vi "AIsFIFO.vi"   [LabVIEW 2017]
uses:
  <vilib>/eio/EIONode/EIONode.xnode
  <vilib>/rvi/DataTransferAndStorage/Container/XNode/niFpgaContainer.xnode
  <vilib>/rvi/eio/common/nirviEmuTemplateMethod_errors.vi
  <vilib>/rvi/FIFO/Fifo_Resource/niFpgaFifoEmulationRefIn.vi
diagram:
  n1 = xnode "FPGA I/O Node"() -> ("Mod1/AI0"=w287, "Mod1/AI1"=w284, "Mod1/AI2"=w281, "Mod1/AI3"=w279, "Mod1/AI4"=w275, "Mod1/AI5"=w272, "Mod1/AI6"=w269, "Mod1/AI7"=w266, "Mod1/AI8"=w263, "Mod1/AI9"=w260, "Mod1/AI10"=w257, "Mod1/AI11"=w254, "Mod1/AI12"=w251, "Mod1/AI13"=w248, "Mod1/AI14"=w245, "Mod1/AI15"=w242, "Mod1/AI16"=w239, "Mod1/AI17"=w236, "Mod1/AI18"=w233, "Mod1/AI19"=w230, "Mod1/AI20"=w227, "Mod1/AI21"=w224, "Mod1/AI22"=w221, "Mod1/AI23"=w218, "Mod1/AI24"=w215, "Mod1/AI25"=w212, "Mod1/AI26"=w209, "Mod1/AI27"=w206, "Mod1/AI28"=w203, "Mod1/AI29"=w200, "Mod1/AI30"=w197, "Mod1/AI31"=w194)  [unwired: 32 in, 32 out]
  n2 = xnode ("FIFO Method Node")("Element"=w287, "Timeout"=10, "FIFO (Eingang)"=refnum<k21> "FIFO" ("FIFO In")) -> ("FIFO (Ausgang)"=w285:refnum<k21>)  [unwired: 1 out]
  n3 = xnode ("FIFO Method Node")("Element"=w284, "Timeout"=10, "FIFO (Eingang)"=w285) -> ("FIFO (Ausgang)"=w282:refnum<k21>)  [unwired: 1 out]
  n4 = xnode ("FIFO Method Node")("Element"=w281, "Timeout"=10, "FIFO (Eingang)"=w282) -> ("FIFO (Ausgang)"=w278:refnum<k21>)  [unwired: 1 out]
  n5 = xnode ("FIFO Method Node")("Element"=w279, "Timeout"=10, "FIFO (Eingang)"=w278) -> ("FIFO (Ausgang)"=w276:refnum<k21>)  [unwired: 1 out]
  n6 = xnode ("FIFO Method Node")("Element"=w275, "Timeout"=10, "FIFO (Eingang)"=w276) -> ("FIFO (Ausgang)"=w273:refnum<k21>)  [unwired: 1 out]
  n7 = xnode ("FIFO Method Node")("Element"=w272, "Timeout"=10, "FIFO (Eingang)"=w273) -> ("FIFO (Ausgang)"=w270:refnum<k21>)  [unwired: 1 out]
  n8 = xnode ("FIFO Method Node")("Element"=w269, "Timeout"=10, "FIFO (Eingang)"=w270) -> ("FIFO (Ausgang)"=w267:refnum<k21>)  [unwired: 1 out]
  n9 = xnode ("FIFO Method Node")("Element"=w266, "Timeout"=10, "FIFO (Eingang)"=w267) -> ("FIFO (Ausgang)"=w264:refnum<k21>)  [unwired: 1 out]
  n10 = xnode ("FIFO Method Node")("Element"=w263, "Timeout"=10, "FIFO (Eingang)"=w264) -> ("FIFO (Ausgang)"=w261:refnum<k21>)  [unwired: 1 out]
  n11 = xnode ("FIFO Method Node")("Element"=w260, "Timeout"=10, "FIFO (Eingang)"=w261) -> ("FIFO (Ausgang)"=w258:refnum<k21>)  [unwired: 1 out]
  n12 = xnode ("FIFO Method Node")("Element"=w257, "Timeout"=10, "FIFO (Eingang)"=w258) -> ("FIFO (Ausgang)"=w255:refnum<k21>)  [unwired: 1 out]
  n13 = xnode ("FIFO Method Node")("Element"=w254, "Timeout"=10, "FIFO (Eingang)"=w255) -> ("FIFO (Ausgang)"=w252:refnum<k21>)  [unwired: 1 out]
  n14 = xnode ("FIFO Method Node")("Element"=w251, "Timeout"=10, "FIFO (Eingang)"=w252) -> ("FIFO (Ausgang)"=w249:refnum<k21>)  [unwired: 1 out]
  n15 = xnode ("FIFO Method Node")("Element"=w248, "Timeout"=10, "FIFO (Eingang)"=w249) -> ("FIFO (Ausgang)"=w246:refnum<k21>)  [unwired: 1 out]
  n16 = xnode ("FIFO Method Node")("Element"=w245, "Timeout"=10, "FIFO (Eingang)"=w246) -> ("FIFO (Ausgang)"=w243:refnum<k21>)  [unwired: 1 out]
  n17 = xnode ("FIFO Method Node")("Element"=w242, "Timeout"=10, "FIFO (Eingang)"=w243) -> ("FIFO (Ausgang)"=w240:refnum<k21>)  [unwired: 1 out]
  n18 = xnode ("FIFO Method Node")("Element"=w239, "Timeout"=10, "FIFO (Eingang)"=w240) -> ("FIFO (Ausgang)"=w237:refnum<k21>)  [unwired: 1 out]
  n19 = xnode ("FIFO Method Node")("Element"=w236, "Timeout"=10, "FIFO (Eingang)"=w237) -> ("FIFO (Ausgang)"=w234:refnum<k21>)  [unwired: 1 out]
  n20 = xnode ("FIFO Method Node")("Element"=w233, "Timeout"=10, "FIFO (Eingang)"=w234) -> ("FIFO (Ausgang)"=w231:refnum<k21>)  [unwired: 1 out]
  n21 = xnode ("FIFO Method Node")("Element"=w230, "Timeout"=10, "FIFO (Eingang)"=w231) -> ("FIFO (Ausgang)"=w228:refnum<k21>)  [unwired: 1 out]
  n22 = xnode ("FIFO Method Node")("Element"=w227, "Timeout"=10, "FIFO (Eingang)"=w228) -> ("FIFO (Ausgang)"=w225:refnum<k21>)  [unwired: 1 out]
  n23 = xnode ("FIFO Method Node")("Element"=w224, "Timeout"=10, "FIFO (Eingang)"=w225) -> ("FIFO (Ausgang)"=w222:refnum<k21>)  [unwired: 1 out]
  n24 = xnode ("FIFO Method Node")("Element"=w221, "Timeout"=10, "FIFO (Eingang)"=w222) -> ("FIFO (Ausgang)"=w219:refnum<k21>)  [unwired: 1 out]
  n25 = xnode ("FIFO Method Node")("Element"=w218, "Timeout"=10, "FIFO (Eingang)"=w219) -> ("FIFO (Ausgang)"=w216:refnum<k21>)  [unwired: 1 out]
  n26 = xnode ("FIFO Method Node")("Element"=w215, "Timeout"=10, "FIFO (Eingang)"=w216) -> ("FIFO (Ausgang)"=w213:refnum<k21>)  [unwired: 1 out]
  n27 = xnode ("FIFO Method Node")("Element"=w212, "Timeout"=10, "FIFO (Eingang)"=w213) -> ("FIFO (Ausgang)"=w210:refnum<k21>)  [unwired: 1 out]
  n28 = xnode ("FIFO Method Node")("Element"=w209, "Timeout"=10, "FIFO (Eingang)"=w210) -> ("FIFO (Ausgang)"=w207:refnum<k21>)  [unwired: 1 out]
  n29 = xnode ("FIFO Method Node")("Element"=w206, "Timeout"=10, "FIFO (Eingang)"=w207) -> ("FIFO (Ausgang)"=w204:refnum<k21>)  [unwired: 1 out]
  n30 = xnode ("FIFO Method Node")("Element"=w203, "Timeout"=10, "FIFO (Eingang)"=w204) -> ("FIFO (Ausgang)"=w201:refnum<k21>)  [unwired: 1 out]
  n31 = xnode ("FIFO Method Node")("Element"=w200, "Timeout"=10, "FIFO (Eingang)"=w201) -> ("FIFO (Ausgang)"=w198:refnum<k21>)  [unwired: 1 out]
  n32 = xnode ("FIFO Method Node")("Element"=w197, "Timeout"=10, "FIFO (Eingang)"=w198) -> ("FIFO (Ausgang)"=w195:refnum<k21>)  [unwired: 1 out]
  n33 = xnode ("FIFO Method Node")("Element"=w194, "Timeout"=10, "FIFO (Eingang)"=w195) -> ("FIFO (Ausgang)"=w97:refnum<k21>)  [unwired: 1 out]
  n34 = xnode "FPGA I/O Node"() -> ("Mod2/AI0"=w191:fxp<+/-,26,5>, "Mod2/AI1"=w188:fxp<+/-,26,5>, "Mod2/AI2"=w185:fxp<+/-,26,5>, "Mod2/AI3"=w183:fxp<+/-,26,5>, "Mod2/AI4"=w179:fxp<+/-,26,5>, "Mod2/AI5"=w176:fxp<+/-,26,5>, "Mod2/AI6"=w173:fxp<+/-,26,5>, "Mod2/AI7"=w170:fxp<+/-,26,5>, "Mod2/AI8"=w167:fxp<+/-,26,5>, "Mod2/AI9"=w164:fxp<+/-,26,5>, "Mod2/AI10"=w161:fxp<+/-,26,5>, "Mod2/AI11"=w158:fxp<+/-,26,5>, "Mod2/AI12"=w155:fxp<+/-,26,5>, "Mod2/AI13"=w152:fxp<+/-,26,5>, "Mod2/AI14"=w149:fxp<+/-,26,5>, "Mod2/AI15"=w146:fxp<+/-,26,5>, "Mod2/AI16"=w143:fxp<+/-,26,5>, "Mod2/AI17"=w140:fxp<+/-,26,5>, "Mod2/AI18"=w137:fxp<+/-,26,5>, "Mod2/AI19"=w134:fxp<+/-,26,5>, "Mod2/AI20"=w131:fxp<+/-,26,5>, "Mod2/AI21"=w128:fxp<+/-,26,5>, "Mod2/AI22"=w125:fxp<+/-,26,5>, "Mod2/AI23"=w122:fxp<+/-,26,5>, "Mod2/AI24"=w119:fxp<+/-,26,5>, "Mod2/AI25"=w116:fxp<+/-,26,5>, "Mod2/AI26"=w113:fxp<+/-,26,5>, "Mod2/AI27"=w110:fxp<+/-,26,5>, "Mod2/AI28"=w107:fxp<+/-,26,5>, "Mod2/AI29"=w104:fxp<+/-,26,5>, "Mod2/AI30"=w101:fxp<+/-,26,5>, "Mod2/AI31"=w98:fxp<+/-,26,5>)  [unwired: 32 in, 32 out]
  n35 = xnode ("FIFO Method Node")("Element"=w191, "Timeout"=10, "FIFO (Eingang)"=w97) -> ("FIFO (Ausgang)"=w189:refnum<k21>)  [unwired: 1 out]
  n36 = xnode ("FIFO Method Node")("Element"=w188, "Timeout"=10, "FIFO (Eingang)"=w189) -> ("FIFO (Ausgang)"=w186:refnum<k21>)  [unwired: 1 out]
  n37 = xnode ("FIFO Method Node")("Element"=w185, "Timeout"=10, "FIFO (Eingang)"=w186) -> ("FIFO (Ausgang)"=w182:refnum<k21>)  [unwired: 1 out]
  n38 = xnode ("FIFO Method Node")("Element"=w183, "Timeout"=10, "FIFO (Eingang)"=w182) -> ("FIFO (Ausgang)"=w180:refnum<k21>)  [unwired: 1 out]
  n39 = xnode ("FIFO Method Node")("Element"=w179, "Timeout"=10, "FIFO (Eingang)"=w180) -> ("FIFO (Ausgang)"=w177:refnum<k21>)  [unwired: 1 out]
  n40 = xnode ("FIFO Method Node")("Element"=w176, "Timeout"=10, "FIFO (Eingang)"=w177) -> ("FIFO (Ausgang)"=w174:refnum<k21>)  [unwired: 1 out]
  n41 = xnode ("FIFO Method Node")("Element"=w173, "Timeout"=10, "FIFO (Eingang)"=w174) -> ("FIFO (Ausgang)"=w171:refnum<k21>)  [unwired: 1 out]
  n42 = xnode ("FIFO Method Node")("Element"=w170, "Timeout"=10, "FIFO (Eingang)"=w171) -> ("FIFO (Ausgang)"=w168:refnum<k21>)  [unwired: 1 out]
  n43 = xnode ("FIFO Method Node")("Element"=w167, "Timeout"=10, "FIFO (Eingang)"=w168) -> ("FIFO (Ausgang)"=w165:refnum<k21>)  [unwired: 1 out]
  n44 = xnode ("FIFO Method Node")("Element"=w164, "Timeout"=10, "FIFO (Eingang)"=w165) -> ("FIFO (Ausgang)"=w162:refnum<k21>)  [unwired: 1 out]
  n45 = xnode ("FIFO Method Node")("Element"=w161, "Timeout"=10, "FIFO (Eingang)"=w162) -> ("FIFO (Ausgang)"=w159:refnum<k21>)  [unwired: 1 out]
  n46 = xnode ("FIFO Method Node")("Element"=w158, "Timeout"=10, "FIFO (Eingang)"=w159) -> ("FIFO (Ausgang)"=w156:refnum<k21>)  [unwired: 1 out]
  n47 = xnode ("FIFO Method Node")("Element"=w155, "Timeout"=10, "FIFO (Eingang)"=w156) -> ("FIFO (Ausgang)"=w153:refnum<k21>)  [unwired: 1 out]
  n48 = xnode ("FIFO Method Node")("Element"=w152, "Timeout"=10, "FIFO (Eingang)"=w153) -> ("FIFO (Ausgang)"=w150:refnum<k21>)  [unwired: 1 out]
  n49 = xnode ("FIFO Method Node")("Element"=w149, "Timeout"=10, "FIFO (Eingang)"=w150) -> ("FIFO (Ausgang)"=w147:refnum<k21>)  [unwired: 1 out]
  n50 = xnode ("FIFO Method Node")("Element"=w146, "Timeout"=10, "FIFO (Eingang)"=w147) -> ("FIFO (Ausgang)"=w144:refnum<k21>)  [unwired: 1 out]
  n51 = xnode ("FIFO Method Node")("Element"=w143, "Timeout"=10, "FIFO (Eingang)"=w144) -> ("FIFO (Ausgang)"=w141:refnum<k21>)  [unwired: 1 out]
  n52 = xnode ("FIFO Method Node")("Element"=w140, "Timeout"=10, "FIFO (Eingang)"=w141) -> ("FIFO (Ausgang)"=w138:refnum<k21>)  [unwired: 1 out]
  n53 = xnode ("FIFO Method Node")("Element"=w137, "Timeout"=10, "FIFO (Eingang)"=w138) -> ("FIFO (Ausgang)"=w135:refnum<k21>)  [unwired: 1 out]
  n54 = xnode ("FIFO Method Node")("Element"=w134, "Timeout"=10, "FIFO (Eingang)"=w135) -> ("FIFO (Ausgang)"=w132:refnum<k21>)  [unwired: 1 out]
  n55 = xnode ("FIFO Method Node")("Element"=w131, "Timeout"=10, "FIFO (Eingang)"=w132) -> ("FIFO (Ausgang)"=w129:refnum<k21>)  [unwired: 1 out]
  n56 = xnode ("FIFO Method Node")("Element"=w128, "Timeout"=10, "FIFO (Eingang)"=w129) -> ("FIFO (Ausgang)"=w126:refnum<k21>)  [unwired: 1 out]
  n57 = xnode ("FIFO Method Node")("Element"=w125, "Timeout"=10, "FIFO (Eingang)"=w126) -> ("FIFO (Ausgang)"=w123:refnum<k21>)  [unwired: 1 out]
  n58 = xnode ("FIFO Method Node")("Element"=w122, "Timeout"=10, "FIFO (Eingang)"=w123) -> ("FIFO (Ausgang)"=w120:refnum<k21>)  [unwired: 1 out]
  n59 = xnode ("FIFO Method Node")("Element"=w119, "Timeout"=10, "FIFO (Eingang)"=w120) -> ("FIFO (Ausgang)"=w117:refnum<k21>)  [unwired: 1 out]
  n60 = xnode ("FIFO Method Node")("Element"=w116, "Timeout"=10, "FIFO (Eingang)"=w117) -> ("FIFO (Ausgang)"=w114:refnum<k21>)  [unwired: 1 out]
  n61 = xnode ("FIFO Method Node")("Element"=w113, "Timeout"=10, "FIFO (Eingang)"=w114) -> ("FIFO (Ausgang)"=w111:refnum<k21>)  [unwired: 1 out]
  n62 = xnode ("FIFO Method Node")("Element"=w110, "Timeout"=10, "FIFO (Eingang)"=w111) -> ("FIFO (Ausgang)"=w108:refnum<k21>)  [unwired: 1 out]
  n63 = xnode ("FIFO Method Node")("Element"=w107, "Timeout"=10, "FIFO (Eingang)"=w108) -> ("FIFO (Ausgang)"=w105:refnum<k21>)  [unwired: 1 out]
  n64 = xnode ("FIFO Method Node")("Element"=w104, "Timeout"=10, "FIFO (Eingang)"=w105) -> ("FIFO (Ausgang)"=w102:refnum<k21>)  [unwired: 1 out]
  n65 = xnode ("FIFO Method Node")("Element"=w101, "Timeout"=10, "FIFO (Eingang)"=w102) -> ("FIFO (Ausgang)"=w99:refnum<k21>)  [unwired: 1 out]
  n66 = xnode ("FIFO Method Node")("Element"=w98, "Timeout"=10, "FIFO (Eingang)"=w99) -> ("FIFO (Ausgang)"=w1:refnum<k21>)  [unwired: 1 out]
  n67 = xnode "FPGA I/O Node"() -> ("Mod3/AI0"=w95, "Mod3/AI1"=w92, "Mod3/AI2"=w89, "Mod3/AI3"=w87, "Mod3/AI4"=w83, "Mod3/AI5"=w80, "Mod3/AI6"=w77, "Mod3/AI7"=w74, "Mod3/AI8"=w71, "Mod3/AI9"=w68, "Mod3/AI10"=w65, "Mod3/AI11"=w62, "Mod3/AI12"=w59, "Mod3/AI13"=w56, "Mod3/AI14"=w53, "Mod3/AI15"=w50, "Mod3/AI16"=w47, "Mod3/AI17"=w44, "Mod3/AI18"=w41, "Mod3/AI19"=w38, "Mod3/AI20"=w35, "Mod3/AI21"=w32, "Mod3/AI22"=w29, "Mod3/AI23"=w26, "Mod3/AI24"=w23, "Mod3/AI25"=w20, "Mod3/AI26"=w17, "Mod3/AI27"=w14, "Mod3/AI28"=w11, "Mod3/AI29"=w8, "Mod3/AI30"=w5, "Mod3/AI31"=w2)  [unwired: 32 in, 32 out]
  n68 = xnode ("FIFO Method Node")("Element"=w95, "Timeout"=10, "FIFO (Eingang)"=w1) -> ("FIFO (Ausgang)"=w93:refnum<k21>)  [unwired: 1 out]
  n69 = xnode ("FIFO Method Node")("Element"=w92, "Timeout"=10, "FIFO (Eingang)"=w93) -> ("FIFO (Ausgang)"=w90:refnum<k21>)  [unwired: 1 out]
  n70 = xnode ("FIFO Method Node")("Element"=w89, "Timeout"=10, "FIFO (Eingang)"=w90) -> ("FIFO (Ausgang)"=w86:refnum<k21>)  [unwired: 1 out]
  n71 = xnode ("FIFO Method Node")("Element"=w87, "Timeout"=10, "FIFO (Eingang)"=w86) -> ("FIFO (Ausgang)"=w84:refnum<k21>)  [unwired: 1 out]
  n72 = xnode ("FIFO Method Node")("Element"=w83, "Timeout"=10, "FIFO (Eingang)"=w84) -> ("FIFO (Ausgang)"=w81:refnum<k21>)  [unwired: 1 out]
  n73 = xnode ("FIFO Method Node")("Element"=w80, "Timeout"=10, "FIFO (Eingang)"=w81) -> ("FIFO (Ausgang)"=w78:refnum<k21>)  [unwired: 1 out]
  n74 = xnode ("FIFO Method Node")("Element"=w77, "Timeout"=10, "FIFO (Eingang)"=w78) -> ("FIFO (Ausgang)"=w75:refnum<k21>)  [unwired: 1 out]
  n75 = xnode ("FIFO Method Node")("Element"=w74, "Timeout"=10, "FIFO (Eingang)"=w75) -> ("FIFO (Ausgang)"=w72:refnum<k21>)  [unwired: 1 out]
  n76 = xnode ("FIFO Method Node")("Element"=w71, "Timeout"=10, "FIFO (Eingang)"=w72) -> ("FIFO (Ausgang)"=w69:refnum<k21>)  [unwired: 1 out]
  n77 = xnode ("FIFO Method Node")("Element"=w68, "Timeout"=10, "FIFO (Eingang)"=w69) -> ("FIFO (Ausgang)"=w66:refnum<k21>)  [unwired: 1 out]
  n78 = xnode ("FIFO Method Node")("Element"=w65, "Timeout"=10, "FIFO (Eingang)"=w66) -> ("FIFO (Ausgang)"=w63:refnum<k21>)  [unwired: 1 out]
  n79 = xnode ("FIFO Method Node")("Element"=w62, "Timeout"=10, "FIFO (Eingang)"=w63) -> ("FIFO (Ausgang)"=w60:refnum<k21>)  [unwired: 1 out]
  n80 = xnode ("FIFO Method Node")("Element"=w59, "Timeout"=10, "FIFO (Eingang)"=w60) -> ("FIFO (Ausgang)"=w57:refnum<k21>)  [unwired: 1 out]
  n81 = xnode ("FIFO Method Node")("Element"=w56, "Timeout"=10, "FIFO (Eingang)"=w57) -> ("FIFO (Ausgang)"=w54:refnum<k21>)  [unwired: 1 out]
  n82 = xnode ("FIFO Method Node")("Element"=w53, "Timeout"=10, "FIFO (Eingang)"=w54) -> ("FIFO (Ausgang)"=w51:refnum<k21>)  [unwired: 1 out]
  n83 = xnode ("FIFO Method Node")("Element"=w50, "Timeout"=10, "FIFO (Eingang)"=w51) -> ("FIFO (Ausgang)"=w48:refnum<k21>)  [unwired: 1 out]
  n84 = xnode ("FIFO Method Node")("Element"=w47, "Timeout"=10, "FIFO (Eingang)"=w48) -> ("FIFO (Ausgang)"=w45:refnum<k21>)  [unwired: 1 out]
  n85 = xnode ("FIFO Method Node")("Element"=w44, "Timeout"=10, "FIFO (Eingang)"=w45) -> ("FIFO (Ausgang)"=w42:refnum<k21>)  [unwired: 1 out]
  n86 = xnode ("FIFO Method Node")("Element"=w41, "Timeout"=10, "FIFO (Eingang)"=w42) -> ("FIFO (Ausgang)"=w39:refnum<k21>)  [unwired: 1 out]
  n87 = xnode ("FIFO Method Node")("Element"=w38, "Timeout"=10, "FIFO (Eingang)"=w39) -> ("FIFO (Ausgang)"=w36:refnum<k21>)  [unwired: 1 out]
  n88 = xnode ("FIFO Method Node")("Element"=w35, "Timeout"=10, "FIFO (Eingang)"=w36) -> ("FIFO (Ausgang)"=w33:refnum<k21>)  [unwired: 1 out]
  n89 = xnode ("FIFO Method Node")("Element"=w32, "Timeout"=10, "FIFO (Eingang)"=w33) -> ("FIFO (Ausgang)"=w30:refnum<k21>)  [unwired: 1 out]
  n90 = xnode ("FIFO Method Node")("Element"=w29, "Timeout"=10, "FIFO (Eingang)"=w30) -> ("FIFO (Ausgang)"=w27:refnum<k21>)  [unwired: 1 out]
  n91 = xnode ("FIFO Method Node")("Element"=w26, "Timeout"=10, "FIFO (Eingang)"=w27) -> ("FIFO (Ausgang)"=w24:refnum<k21>)  [unwired: 1 out]
  n92 = xnode ("FIFO Method Node")("Element"=w23, "Timeout"=10, "FIFO (Eingang)"=w24) -> ("FIFO (Ausgang)"=w21:refnum<k21>)  [unwired: 1 out]
  n93 = xnode ("FIFO Method Node")("Element"=w20, "Timeout"=10, "FIFO (Eingang)"=w21) -> ("FIFO (Ausgang)"=w18:refnum<k21>)  [unwired: 1 out]
  n94 = xnode ("FIFO Method Node")("Element"=w17, "Timeout"=10, "FIFO (Eingang)"=w18) -> ("FIFO (Ausgang)"=w15:refnum<k21>)  [unwired: 1 out]
  n95 = xnode ("FIFO Method Node")("Element"=w14, "Timeout"=10, "FIFO (Eingang)"=w15) -> ("FIFO (Ausgang)"=w12:refnum<k21>)  [unwired: 1 out]
  n96 = xnode ("FIFO Method Node")("Element"=w11, "Timeout"=10, "FIFO (Eingang)"=w12) -> ("FIFO (Ausgang)"=w9:refnum<k21>)  [unwired: 1 out]
  n97 = xnode ("FIFO Method Node")("Element"=w8, "Timeout"=10, "FIFO (Eingang)"=w9) -> ("FIFO (Ausgang)"=w6:refnum<k21>)  [unwired: 1 out]
  n98 = xnode ("FIFO Method Node")("Element"=w5, "Timeout"=10, "FIFO (Eingang)"=w6) -> ("FIFO (Ausgang)"=w3:refnum<k21>)  [unwired: 1 out]
  n99 = xnode ("FIFO Method Node")("Element"=w2, "Timeout"=10, "FIFO (Eingang)"=w3) -> ()  [unwired: 2 out]
